vi "ArduinoLightSwitch_and_TempMonitor-V1 - Copy.vi"(8 "error in":errorcluster, 10 "Spotlights":bool, 11 "Coaxial light":bool) -> (0 "error out":errorcluster, 3 "Thermometer [C]":dbl(slide) scale=0.0..100.0)   [LabVIEW 2016]
uses:
  <vilib>/LabVIEW Interface for Arduino/Type Defs/Pin Mode.ctl
  <vilib>/LabVIEW Interface for Arduino/LabVIEW Interface for Arduino.lvlib
panel:
  in  "Tab Control":T1(tab)
  in  "Digital I/O Pin - Spotlights":u8=6
  in  "Digital I/O Pin - Coaxial":u8=5
  out "VCC [V]":dbl=5.0 format="%#_13g"
  in  "Units (C)":enum16{"Celsius", "Fahrenheit", "Kelvin"}(ring)
  in  "Thermistor Analogue Pin":u8=1
  in  "Paired Resistance (10K Ohms)":dbl=10000.0 format="%#_13g"
  in  "Vcc Reference Analog Input Pin":u8
  in  "VISA resource":refnum<visa-resource-name>
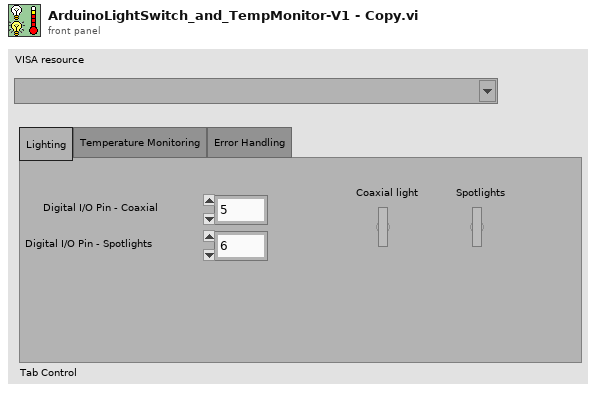
[diagram p1: front panel]
types:
  T1 = enum32{"Lighting", "Temperature Monitoring", "Error Handling"}
  T2 = typedef "LabVIEW Interface for Arduino.lvlib/Pin Mode.ctl" = enum8{"Input", "Output"}
  T3 = typedef "LabVIEW Interface for Arduino.lvlib/Arduino Resource.ctl" = cluster{"VISA resource":refnum<visa-resource-name>, "Board Type":T4, "Connection Type":enum8{"USB / Serial"}, "Bytes Per Packet (15)":u8}
  T4 = typedef "LabVIEW Interface for Arduino.lvlib/Board Type.ctl" = enum16{"Uno", "Dimuelanove w/Atmega 328", "Mega 2560"}
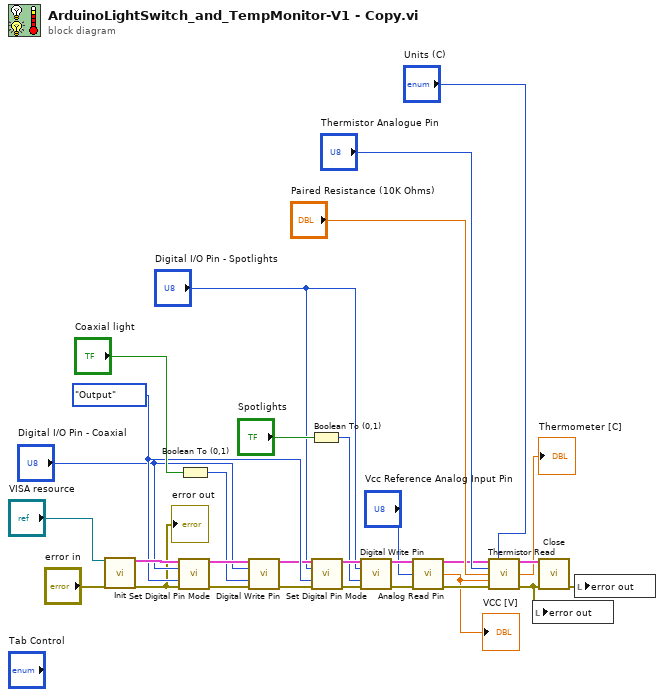
[diagram p0: block diagram]
diagram:
  w16 = Pin_Mode."Output" ("Pin Mode (Input)")
  n1 = call <vilib>:"Init.vi"("VISA resource"="VISA resource", "error in"="error in") -> ("Arduino Resource"=w27:T3, "error out"=w7:errorcluster)  [unwired: 16 in]
  "error out" <- w7
  n2 = call <vilib>:"Set Digital Pin Mode.vi"("Arduino Resource"=w27, "Digital I/O Pin"="Digital I/O Pin - Coaxial", "Pin Mode (Input)"=w16, "error in"=w7) -> ("Arduino Resource"=w21:T3, "error out"=w20:errorcluster)  [unwired: 10 in]
  n3 = Boolean To (0,1)(Boolean="Coaxial light") -> (0, 1=w13:i16)
  n4 = call <vilib>:"Digital Write Pin.vi"("Arduino Resource"=w21, "Digital I/O Pin (0)"="Digital I/O Pin - Coaxial", "Value (0)"=w13, "error in"=w20) -> ("Arduino Resource"=w15:T3, "error out"=w9:errorcluster)  [unwired: 10 in]
  n5 = Boolean To (0,1)(Boolean="Spotlights") -> (0, 1=w12:i16)
  n6 = call <vilib>:"Set Digital Pin Mode.vi"("Arduino Resource"=w15, "Digital I/O Pin"="Digital I/O Pin - Spotlights", "Pin Mode (Input)"=w16, "error in"=w9) -> ("Arduino Resource"=w19:T3, "error out"=w18:errorcluster)  [unwired: 10 in]
  n7 = call <vilib>:"Digital Write Pin.vi"("Arduino Resource"=w19, "Digital I/O Pin (0)"="Digital I/O Pin - Spotlights", "Value (0)"=w12, "error in"=w18) -> ("Arduino Resource"=w6:T3, "error out"=w5:errorcluster)  [unwired: 10 in]
  n8 = call <vilib>:"Analog Read Pin.vi"("Arduino Resource"=w6, "Analog Input Pin (0)"="Vcc Reference Analog Input Pin", "error in"=w5) -> ("Arduino Resource"=w3:T3, "Voltage"=w1:dbl, "error out"=w2:errorcluster)  [unwired: 10 in]
  "VCC [V]" <- w1
  n9 = call <vilib>:"Thermistor Read.vi"("Arduino Resource"=w3, "Units (C)"="Units (C)", "Thermistor AI Pin (0)"="Thermistor Analogue Pin", "Paired Resistance (10K Ohms)"="Paired Resistance (10K Ohms)", "Vcc (5 v)"=w1, "error in"=w2) -> ("Arduino Resource"=w26:T3, "Temperature"=→"Thermometer [C]":dbl, "error out"=w25:errorcluster)  [unwired: 7 in]
  n10 = local write "error out"(w25) -> ()
  n11 = call <vilib>:"Close.vi"("Arduino Resource"=w26, "error in"=w25) -> ("error out"=w28:errorcluster)  [unwired: 13 in]
  n12 = local write "error out"(w28) -> ()
